vi "SimpleBalanceAndControl 26th April.vi"() -> ()   [LabVIEW 2021]
uses:
  <vilib>/addons/control/pid/pid.llb/PID (DBL).vi
  <vilib>/addons/control/pid/NI_PID_pid.lvlib
panel:
  out "Contact time ms":sgl format="%#_8g"
  out "Ball in grabbed":bool
  out "Ball out of contact":bool
  out "Contact":bool
  out "R_Claw":bool
  out "L_Claw":bool
  out "Ball_cs":bool
  in  "On/Off":bool
  in  "Speed":sgl
  in  "Claw direction":bool
  out "String":string
  in  "Forward":bool
  in  "Backward":bool
  in  "Left":bool
  in  "Right":bool
  out "Control Data":T1(graph)
  out "Error":dbl
  in  "setpoint":sgl format="%.2f"
  in  "PID gains":T2={"proportional gain (Kc)"=1.0, "integral time (Ti, min)"=0.01, "derivative time (Td, min)"=0.0} {"derivative time (Td, min)" format="%.8f"; "integral time (Ti, min)" format="%.8f"; "proportional gain (Kc)" format="%.8f"}
  in  "output range":cluster{"output high":dbl, "output low":dbl}={"output high"=100.0, "output low"=-100.0} {"output low" format="%.2f"; "output high" format="%.2f"}
  out "Waveform IMU":T3(graph)
  out "AngleZ":sgl
  out "AngleY":sgl
  out "AngleX":sgl
  in  "stop":bool
  # "Down = Open"
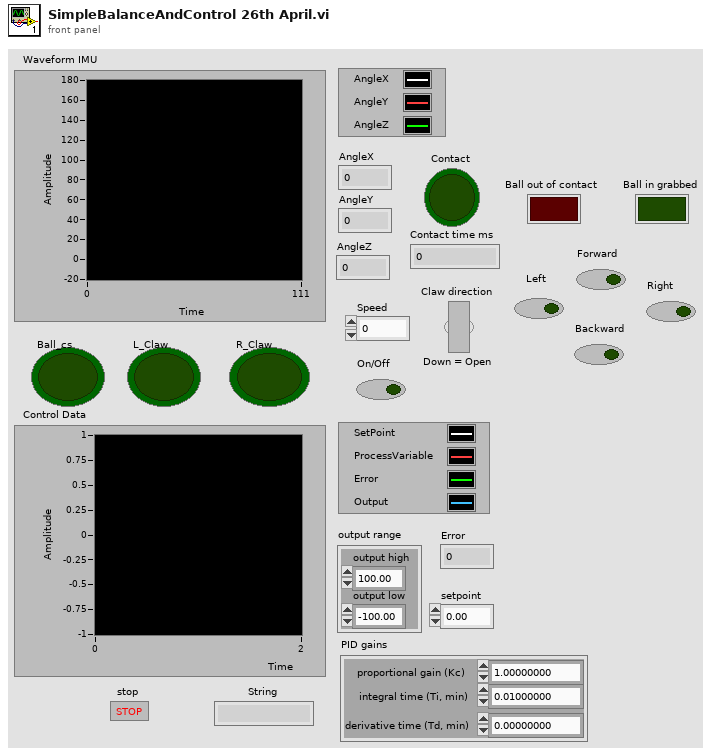
[diagram p1: front panel]
types:
  T1 = cluster{"setpoint":sgl, "bytes to read":sgl, "Error":sgl, "output":sgl}
  T2 = cluster{"proportional gain (Kc)":dbl, "integral time (Ti, min)":dbl, "derivative time (Td, min)":dbl}
  T3 = cluster{"bytes to read":sgl, "bytes to read":sgl, "bytes to read":sgl}
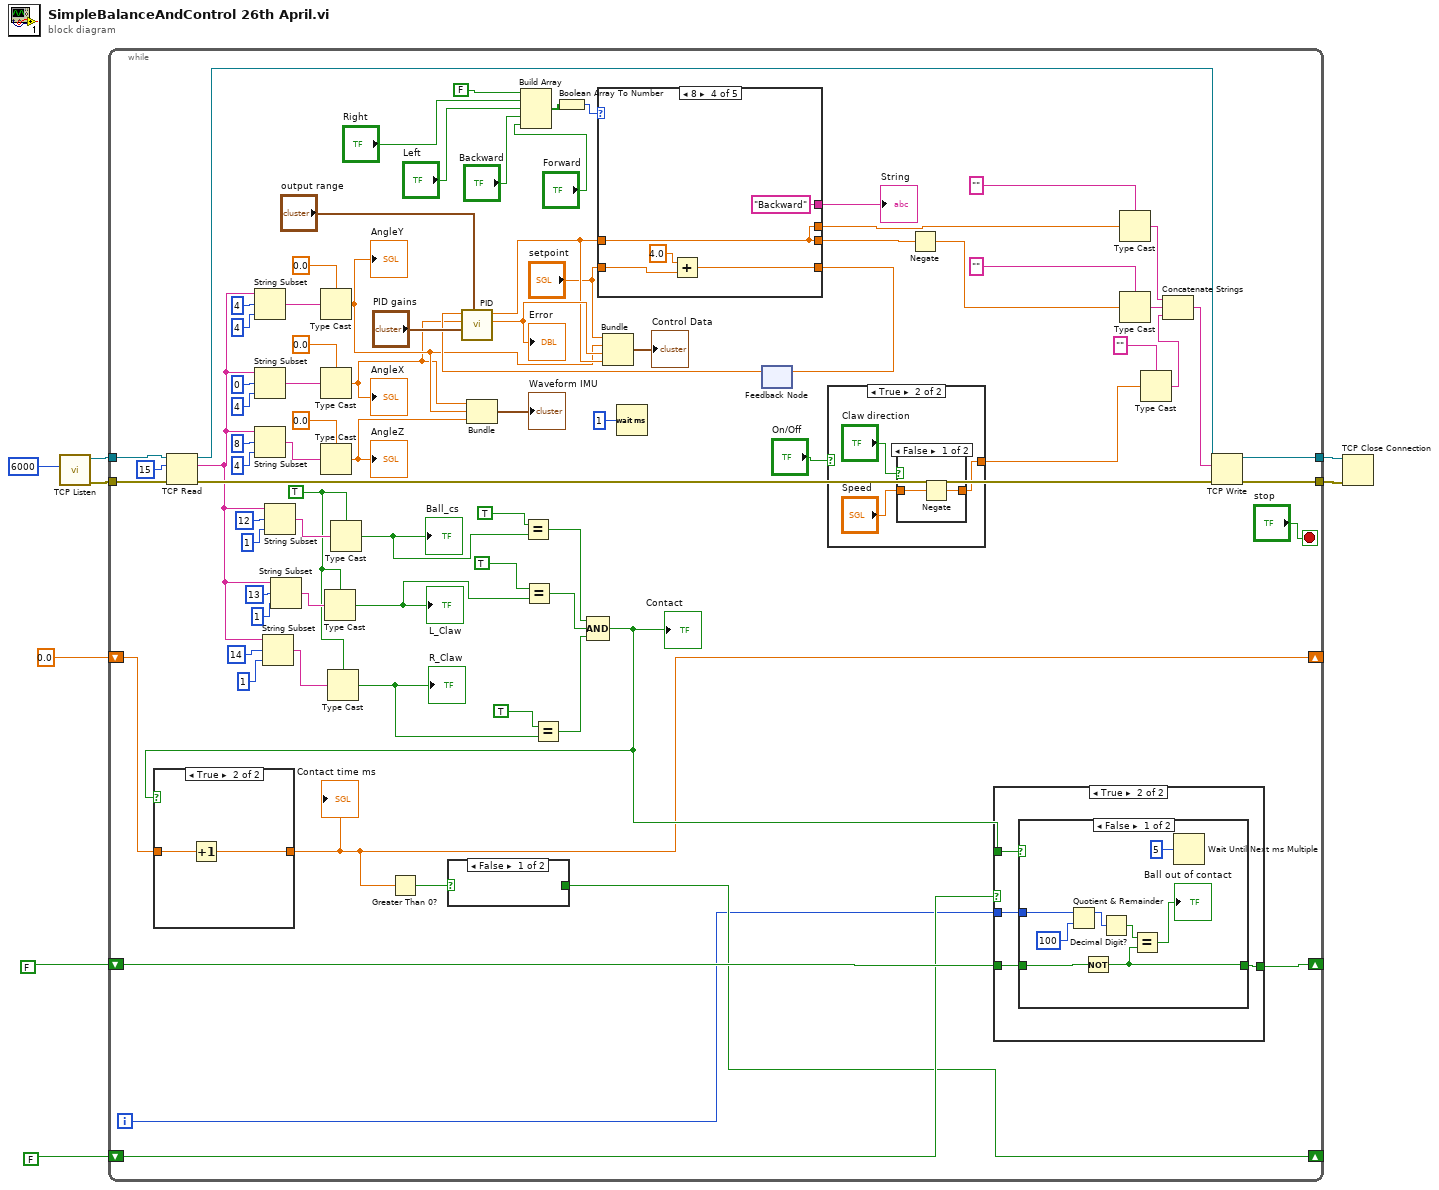
[diagram p0: block diagram]
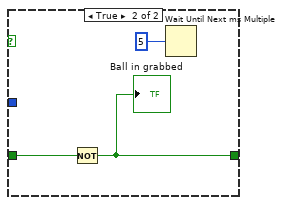
[diagram p4: hidden frame]
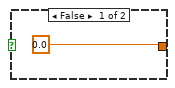
[diagram p6: hidden frame]
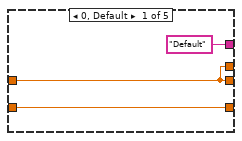
[diagram p8: hidden frame]
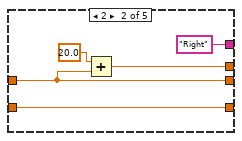
[diagram p9: hidden frame]
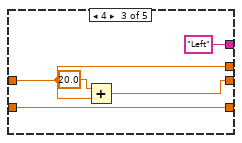
[diagram p10: hidden frame]
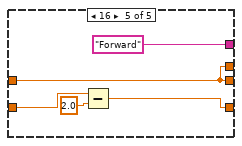
[diagram p11: hidden frame]
diagram:
  n1 = call <vilib>:"TCP Listen.vi"("port"=u16 6000) -> ("error out"=w7:errorcluster, "connection ID"=w8:refnum<k5>)  [unwired: 6 in, 3 out]
  n2 = while {
    tunnel: w8 -> [w88]
    tunnel: w7 -> [w87]
    tunnel: [w69] -> w5
    tunnel: [w68] -> w4
    shift-right: [w12] -> _
    shift-left: sgl 0.0 -> [w17]
    shift-right: [w15] -> _
    shift-left: FALSE -> [w16]
    shift-right: [w10] -> _
    shift-left: FALSE -> [w14]
    i -> [w9]
    stop <- "stop" stop-if-true
    w27 = TRUE
    n3 = TCP Read(connection ID=w88, bytes to read=15, error in (no error)=w87) -> (connection ID out=w71:refnum<k5>, data out=w28:string, error out=w70:errorcluster)  [unwired: 2 in]
    n4 = String Subset(string=w28, offset (0)=4, length (rest)=4 ("length (rest)")) -> (substring=w81:string)
    n5 = String Subset(string=w28, offset (0)=0, length (rest)=4 ("length (rest)")) -> (substring=w82:string)
    n6 = String Subset(string=w28, offset (0)=8, length (rest)=4 ("length (rest)")) -> (substring=w80:string)
    n7 = String Subset(string=w28, offset (0)=14, length (rest)=1 ("length (rest)")) -> (substring=w31:string)
    n8 = String Subset(string=w28, offset (0)=12, length (rest)=1 ("length (rest)")) -> (substring=w37:string)
    n9 = String Subset(string=w28, offset (0)=13, length (rest)=1 ("length (rest)")) -> (substring=w34:string)
    n10 = Type Cast(type=sgl 0.0 ("bytes to read"), x=w81) -> (*(type *) &x=w46:sgl)
    "AngleY" <- w46
    n11 = Type Cast(type=sgl 0.0 ("bytes to read"), x=w82) -> (*(type *) &x=w45:sgl)
    "AngleX" <- w45
    n12 = Type Cast(type=sgl 0.0 ("bytes to read"), x=w80) -> (*(type *) &x=w73:sgl)
    "AngleZ" <- w73
    n13 = Type Cast(type=w27, x=w34) -> (*(type *) &x=w24:bool)
    "L_Claw" <- w24
    n14 = Type Cast(type=w27, x=w31) -> (*(type *) &x=w18:bool)
    "R_Claw" <- w18
    n15 = Type Cast(type=w27, x=w37) -> (*(type *) &x=w22:bool)
    "Ball_cs" <- w22
    n16 = Bundle("bytes to read"=w45, "bytes to read"=w46, "bytes to read"=w73) -> (→"Waveform IMU":T3)  [unwired: 1 in]
    n17 = Build Array(FALSE ("element"), "Right", "Left", "Backward", "Forward") -> (w57:bool[])
    n18 = Equal?(x=TRUE, y=w22) -> (x = y?=w21:bool)
    n19 = Equal?(x=TRUE, y=w24) -> (x = y?=w20:bool)
    n20 = Equal?(x=TRUE, y=w18) -> (x = y?=w19:bool)
    n21 = Boolean Array To Number(Boolean array=w57) -> (number=w58:u32)
    n22 = Compound Arithmetic op=AND(w21, w20, w19) -> (w13:bool)
    "Contact" <- w13
    n23 = case shown="True" w13 {
      tunnel: [w107 w108] -> w12
      tunnel: w17 -> [w107 w109]
      frame False {
      }
      frame True {
        n24 = Increment(x=w109) -> (x+1=w108:sgl)
      }
    }
    "Contact time ms" <- w12
    n25 = Greater Than 0?(x=w12) -> (x > 0?=w11:bool)
    n26 = case shown="False" w11 {
      selector: w11 -> [_ w91]
      tunnel: [_ w91] -> w10
      frame False {
      }
      frame True {
      }
    }
    n27 = Wait (ms)(milliseconds to wait=u32 1) -> ()  [unwired: 1 out]
    n28 = feedback #1() -> (w48:sgl)  [unwired: 1 in]
    n29 = call-poly <vilib>:"PID.vi"("output range"="output range", "PID gains"="PID gains", "process variable"=w45, "setpoint"=w48) -> ("Error"=w61:sgl, "output"=w51:sgl)  [unwired: 5 in, 1 out]
    "Error" <- w61
    n30 = case shown="8" w58 {
      tunnel: w51 -> [w119 w123 w128 w134 w136]
      tunnel: [w119 w122 w128 w134 w136] -> w44
      tunnel: [w119 w123 w129 w134 w136] -> w43
      tunnel: "setpoint" -> [w118 w121 w126 w132 w139]
      tunnel: [w118 w121 w126 w131 w138] -> w49
      tunnel: ["Default" "Right" "Left" "Backward" "Forward"] -> w47
      frame 0, Default {
      }
      frame 2 {
        n31 = Add(x=sgl 20.0, y=w123) -> (x+y=w122:sgl)
      }
      frame 4 {
        n32 = Add(x=sgl 20.0, y=w128) -> (x+y=w129:sgl)
      }
      frame 8 {
        n33 = Add(x=sgl 4.0, y=w132) -> (x+y=w131:sgl)
      }
      frame 16 {
        n34 = Subtract(x=w139, y=sgl 2.0) -> (x-y=w138:sgl)
      }
    }
    "String" <- w47
    n35 = Bundle("setpoint"="setpoint", "bytes to read"=w46, "Error"=w61, "output"=w51) -> (→"Control Data":T1)  [unwired: 1 in]
    n36 = feedback-in #1(w49) -> ()
    n37 = case shown="True" "On/Off" {
      tunnel: [sgl 0.0 w113] -> w39
      frame False {
      }
      frame True {
        n38 = case shown="False" "Claw direction" {
          tunnel: "Speed" -> [w114 w116]
          tunnel: [w115 w116] -> w113
          frame False {
            n39 = Negate(x=w114) -> (-x=w115:sgl)
          }
          frame True {
          }
        }
      }
    }
    n40 = Negate(x=w43) -> (-x=w42:sgl)
    n41 = case shown="True" w14 {
      tunnel: w16 -> [_ w95]
      tunnel: [_ w94] -> w15
      tunnel: w13 -> [_ w93]
      tunnel: w9 -> [_ w92]
      frame False {
      }
      frame True {
        n42 = case shown="False" w93 {
          tunnel: w95 -> [w102 w106]
          tunnel: [w98 w105] -> w94
          tunnel: w92 -> [w101 _]
          frame False {
            n43 = Quotient & Remainder(x=w101, y=100) -> (x-y*floor(x/y)=w96:i32)  [unwired: 1 out]
            n44 = Not(x=w102) -> (.not. x?=w98:bool)
            n45 = Decimal Digit?(1:w96) -> (0:w99:bool)
            n46 = Equal?(x=w99, y=w98) -> (x = y?=→"Ball out of contact":bool)
            n47 = Wait Until Next ms Multiple(millisecond multiple=u32 5) -> ()  [unwired: 1 out]
          }
          frame True {
            n48 = Not(x=w106) -> (.not. x?=w105:bool)
            "Ball in grabbed" <- w105
            n49 = Wait Until Next ms Multiple(millisecond multiple=u32 5) -> ()  [unwired: 1 out]
          }
        }
      }
    }
    n50 = Type Cast(type="", x=w44) -> (*(type *) &x=w66:string)
    n51 = Type Cast(type="", x=w42) -> (*(type *) &x=w65:string)
    n52 = Type Cast(type="", x=w39) -> (*(type *) &x=w40:string)
    n53 = Concatenate Strings(w66, w65, w40) -> (w64:string)
    n54 = TCP Write(connection ID=w71, data in=w64, error in (no error)=w70) -> (connection ID out=w68:refnum<k5>, error out=w69:errorcluster)  [unwired: 1 in, 1 out]
  }
  n55 = TCP Close Connection(connection ID=w4, error in (no error)=w5) -> ()  [unwired: 1 in, 2 out]
